vi "Get Serial Data.vi"(11 "SerialIO":refnum<class "Alicat Device.lvclass">[](array[class])) -> (0 "error out":errorcluster, 1 "flows":sgl[](array[numeric]), 2 "purge":sgl, 3 "DataOut":refnum<class "Data.lvclass">[](array[class]))   [LabVIEW 2015, in "cCRDS.lvclass"]
doc: "Retrieve the Alicat data which will be returned in the <b>DataOut</b> array of Data objects. The data will also be pumped out in an array of clusters for processing in the <b>Get Data</b> method of the cCRDS class."
uses:
  cCRDS.lvclass
  Reusable/Data/Data.lvclass
  Devices/Alicat/Session Based/Alicat Device.lvclass
  Devices/Alicat/Session Based/Data/Alicat Data.lvclass
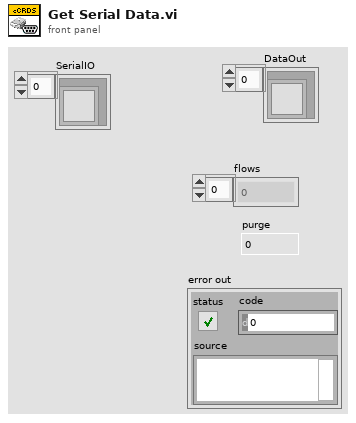
[diagram p1: front panel]
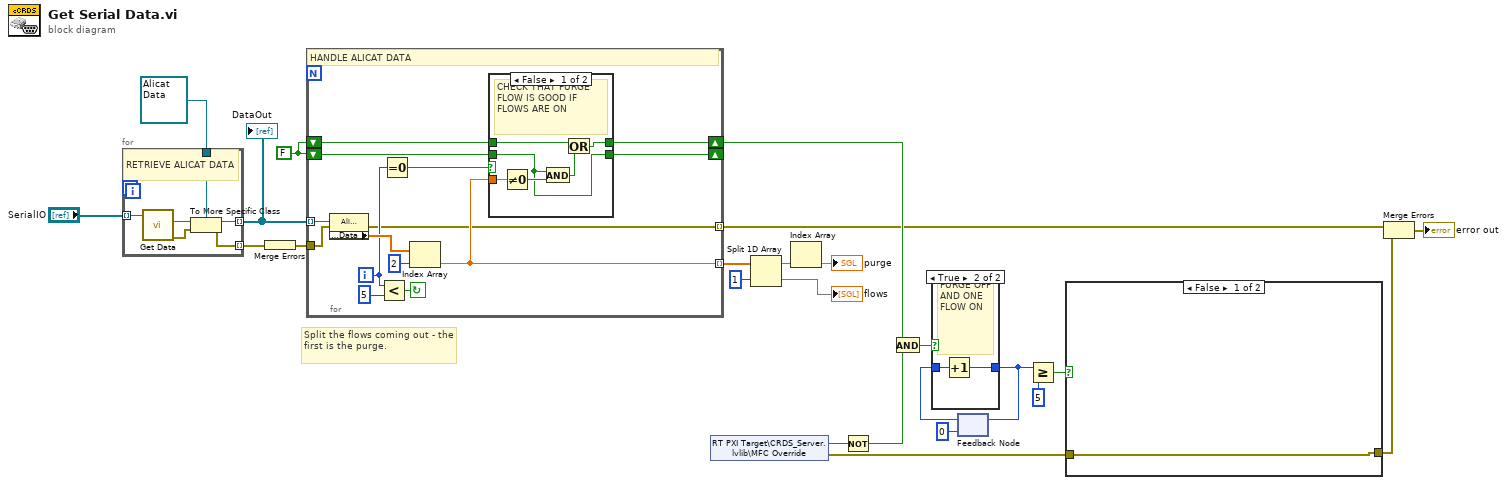
[diagram p0: block diagram]
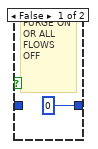
[diagram p2: hidden frame]
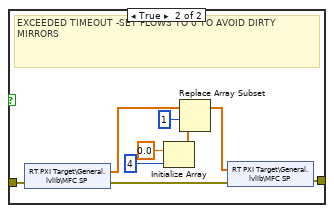
[diagram p3: hidden frame]
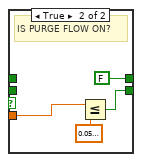
[diagram p4: hidden frame]
diagram:
  w14 = FALSE
  # "Split the flows coming out - the first is the purge."
  n1 = for {
    tunnel: "SerialIO" -> [w30] mode=indexing
    tunnel: [w25] -> w22 mode=indexing
    tunnel: [w27] -> w2 mode=indexing
    tunnel: refnum<class "Alicat Data.lvclass"> refnum ("Alicat Data") -> [w28]
    # "RETRIEVE ALICAT DATA"
    n2 = call-dynamic "Get Data.vi"("Cfg Dev in"=w30) -> ("error out"=w26:errorcluster, "DataOut"=w29:refnum<class "Data.lvclass">)  [unwired: 8 in, 1 out]
    n3 = To More Specific Class(target class=w28, reference=w29, error in=w26) -> (specific class reference=w27:refnum<class "Alicat Data.lvclass">, error out=w25:errorcluster)
  }
  "DataOut" <- w2
  n4 = Merge Errors(w22) -> (w23:errorcluster)
  n5 = for {
    tunnel: w2 -> [w36] mode=indexing
    tunnel: w23 -> [w37]
    tunnel: [w31] -> w11 mode=indexing
    shift-right: [w41] -> _
    shift-left: w14 -> [w40]
    shift-right: [w39] -> w13
    shift-left: w14 -> [w38]
    tunnel: [w32] -> w7 mode=indexing
    i -> [w33]
    stop <- w43 continue-if-true
    # "HANDLE ALICAT DATA"
    n6 = property class="Alicat Data"(reference=w36, error in=w37) -> (error out=w31:errorcluster, "Accessors:Data"=w35:sgl[])  [unwired: 1 out]
    n7 = Less?(x=w33, y=5) -> (x < y?=w43:bool)
    n8 = Equal To 0?(x=w33) -> (x = 0?=w42:bool)
    n9 = Index Array(array=w35, index=2) -> (element=w32:sgl)
    n10 = case shown="False" w42 {
      tunnel: w32 -> [w50 w53]
      tunnel: [w45 w52] -> w41
      tunnel: w40 -> [w45 _]
      tunnel: [w48 FALSE] -> w39
      tunnel: w38 -> [w47 _]
      frame False {
        # "CHECK THAT PURGE FLOW IS GOOD IF FLOWS ARE ON"
        n11 = Not Equal To 0?(x=w50) -> (x != 0?=w49:bool)
        n12 = And(x=w45, y=w49) -> (x .and. y?=w46:bool)
        n13 = Or(x=w47, y=w46) -> (x .or. y?=w48:bool)
      }
      frame True {
        # "IS PURGE FLOW ON?"
        n14 = Less Or Equal?(x=w53, y=sgl 0.05) -> (x <= y?=w52:bool)
      }
    }
  }
  n15 = shared-variable "RT PXI Target\\CRDS_Server.lvlib\\MFC Override"() -> (w17:bool, error out=w8:errorcluster)  [unwired: 1 in]
  n16 = Split 1D Array(array=w7, index=1) -> (first subarray=w5:sgl[], second subarray=→"flows":sgl[])
  n17 = Index Array(array=w5) -> (element=→"purge":sgl)  [unwired: 1 in]
  n18 = Not(x=w17) -> (.not. x?=w16:bool)
  n19 = And(x=w13, y=w16) -> (x .and. y?=w15:bool)
  n20 = feedback #1(0) -> (w20:i32)
  n21 = case shown="True" w15 {
    tunnel: [0 w56] -> w19
    tunnel: w20 -> [_ w57]
    frame False {
      # "PURGE ON OR ALL FLOWS OFF"
    }
    frame True {
      # "PURGE OFF AND ONE FLOW ON"
      n22 = Increment(x=w57) -> (x+1=w56:i32)
    }
  }
  n23 = feedback-in #1(w19) -> ()
  n24 = Greater Or Equal?(x=w19, y=5) -> (x >= y?=w12:bool)
  n25 = case shown="False" w12 {
    tunnel: [w58 w60] -> w10
    tunnel: w8 -> [w58 w59]
    frame False {
    }
    frame True {
      # "EXCEEDED TIMEOUT -SET FLOWS TO 0 TO AVOID DIRTY MIRRORS"
      n26 = shared-variable "RT PXI Target\\General.lvlib\\MFC SP"(error in=w59) -> (w66:sgl[], error out=w67:errorcluster)
      n27 = Initialize Array(sgl 0.0 ("element"), 4 ("dimension size")) -> (w61:sgl[])
      n28 = Replace Array Subset(array=w66, new element=w61, index=1) -> (w64:sgl[])
      n29 = shared-variable "RT PXI Target\\General.lvlib\\MFC SP"(w64, error in=w67) -> (error out=w60:errorcluster)
    }
  }
  n30 = Merge Errors(w11, w10) -> (→"error out":errorcluster)
